vi "Find Available EndPoint.vi"(9 "Excludes":string[](array[string])) -> (4 "IPEndPoint":T1, 15 "error out":errorcluster)   [LabVIEW 2020, in "epl-network.lvlib"]
uses:
  epl-network.lvlib
  TCP/Typedefs/IPEndPoint.ctl
panel:
  out "port":u16
  out "address":string
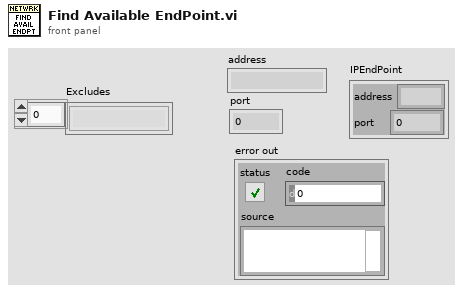
[diagram p1: front panel]
types:
  T1 = typedef "epl-network.lvlib/IPEndPoint.ctl" = cluster{"address":string, "port":i32}
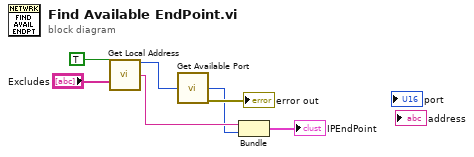
[diagram p0: block diagram]
diagram:
  n1 = call "Get Local Address.vi"("LAN first"=TRUE, "Excludes"="Excludes") -> ("net address"=w5:u32, "address"=w3:string)  [unwired: 12 in]
  n2 = call "Get Available Port.vi"("net address"=w5) -> ("port"=w2:u16, "error out"=→"error out":errorcluster)  [unwired: 13 in]
  n3 = Bundle("address"=w3, "port"=w2) -> (→"IPEndPoint":cluster{"address":string, "port":u16})  [unwired: 1 in]
